vi "Check Authentication.vi"(8 "error in (no error)":errorcluster, 11 "Web Request in":refnum<class "Web Request.lvclass">) -> (0 "error out":errorcluster, 1 "HTTP Status Code":T1={"HTTP Code"=200, "JSON Response"={"error"="No Error", "reason"="No Error"}}, 2 "Logged in?":bool, 3 "Web Request out":refnum<class "Web Request.lvclass">, 5 "Username":string)   [LabVIEW 2016, in "WSsupport.lvlib"]
uses:
  WSsupport.lvlib
  <vilib>/wsapi/Web Request.lvclass
  ServerErrors/Error Message--cluster.ctl
  ServerErrors/ServerErrors.lvlib
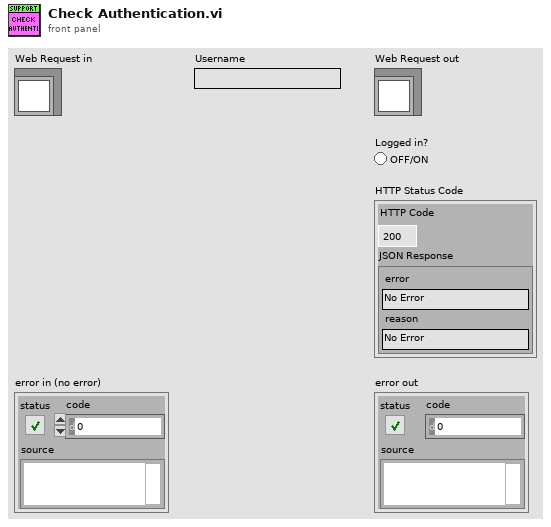
[diagram p1: front panel]
types:
  T1 = typedef "ServerErrors.lvlib/Error Message--cluster.ctl" = cluster{"HTTP Code":i32, "JSON Response":cluster{"error":string, "reason":string}}
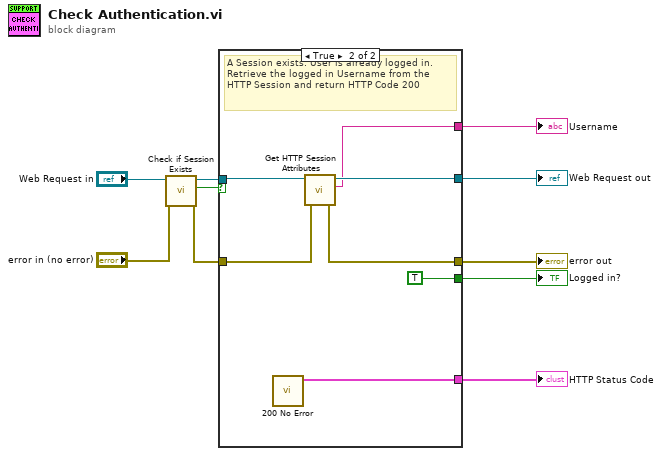
[diagram p0: block diagram]
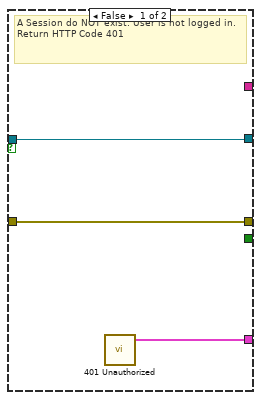
[diagram p2: hidden frame]
diagram:
  n1 = call "Check if Session Exists.vi"("error in (no error)"="error in (no error)", "Web Request in"="Web Request in") -> ("error out"=w6:errorcluster, "Logged in"=w4:bool, "Web Request out"=w5:refnum<class "Web Request.lvclass">)  [unwired: 7 in]
  n2 = case shown="True" w4 {
    tunnel: w5 -> [w11 w16]
    tunnel: w6 -> [w12 w20]
    tunnel: [w13 w19] -> w2
    tunnel: [w12 w17] -> w10
    tunnel: [w11 w15] -> w9
    tunnel: [_ TRUE] -> w8
    tunnel: [_ w14] -> w1
    frame False {
      # "A Session do NOT exist. User is not logged in. Return HTTP Code 401"
      n3 = call "401 Unauthorized.vi"() -> ("error"=w13:T1)  [unwired: 11 in]
    }
    frame True {
      # "A Session exists. User is already logged in. Retrieve the logged in Username from the HTTP Session and return HTTP Code 200"
      n4 = call "200 No Error.vi"() -> ("no error"=w19:T1)  [unwired: 11 in]
      n5 = call "Get HTTP Session Attributes.vi"("error in (no error)"=w20, "Web Request in"=w16) -> ("error out"=w17:errorcluster, "Username"=w14:string, "Web Request out"=w15:refnum<class "Web Request.lvclass">)  [unwired: 7 in]
    }
  }
  "error out" <- w10
  "Web Request out" <- w9
  "Logged in?" <- w8
  "HTTP Status Code" <- w2
  "Username" <- w1
